vi "Filters.vi"() -> ()   [LabVIEW 2009]
uses:
  <vilib>/vision/NI_Vision_Development_Module.lvlib
panel:
  out "Filter Binary":T1(plugin-control)
  in  "file (use dialog)":path=path "C:/Documents and Settings/dgrieneisen/My Documents/Robotics/Athena/weights.fl"
  in  "Stop":bool
  in  "Filter Select":T2(radio)
  out "Filter Settings":T2(tab)
  in  "Red Range":cluster{"Lower value":i32, "Upper value":i32}={"Lower value"=120, "Upper value"=200}
  in  "Green Range":cluster{"Lower value":i32, "Upper value":i32}={"Lower value"=0, "Upper value"=255}
  in  "Blue Range":cluster{"Lower value":i32, "Upper value":i32}={"Lower value"=100, "Upper value"=255}
  in  "Color Mode":u16(ring) items=["RGB", "HSL", "HSV", "HSI"]
  in  "Hue Range":cluster{"Lower value":i32, "Upper value":i32}={"Lower value"=0, "Upper value"=255}
  in  "Saturation Range":cluster{"Lower value":i32, "Upper value":i32}={"Lower value"=0, "Upper value"=255}
  in  "Luma Range":cluster{"Lower value":i32, "Upper value":i32}={"Lower value"=0, "Upper value"=255}
  in  "Color Mode HSL":u16(ring)=1 items=["RGB", "HSL", "HSV", "HSI"]
  in  "Red Scalar":sgl=3.0
  in  "Green Scalar":sgl=3.0
  in  "Blue Scalar":sgl=3.3
  in  "Luma Scalar Low":sgl=4.0
  in  "Sat Scalar":sgl=2.5
  in  "Hue Scalar":sgl=5.0
  in  "Luma Scalar High":sgl=4.0
  in  "res/2":i32=3
  in  "Sample Rate":i32=3
  in  "ANN Level":dbl=0.5
  in  "ANN Out Switch":bool
  in  "Input Image Path":path=path "C:/Documents and Settings/dgrieneisen/My Documents/Robotics/Athena/image2004.jpg"
  out "'input Image":T1(plugin-control)
  out "Filtered Image":T1(plugin-control)
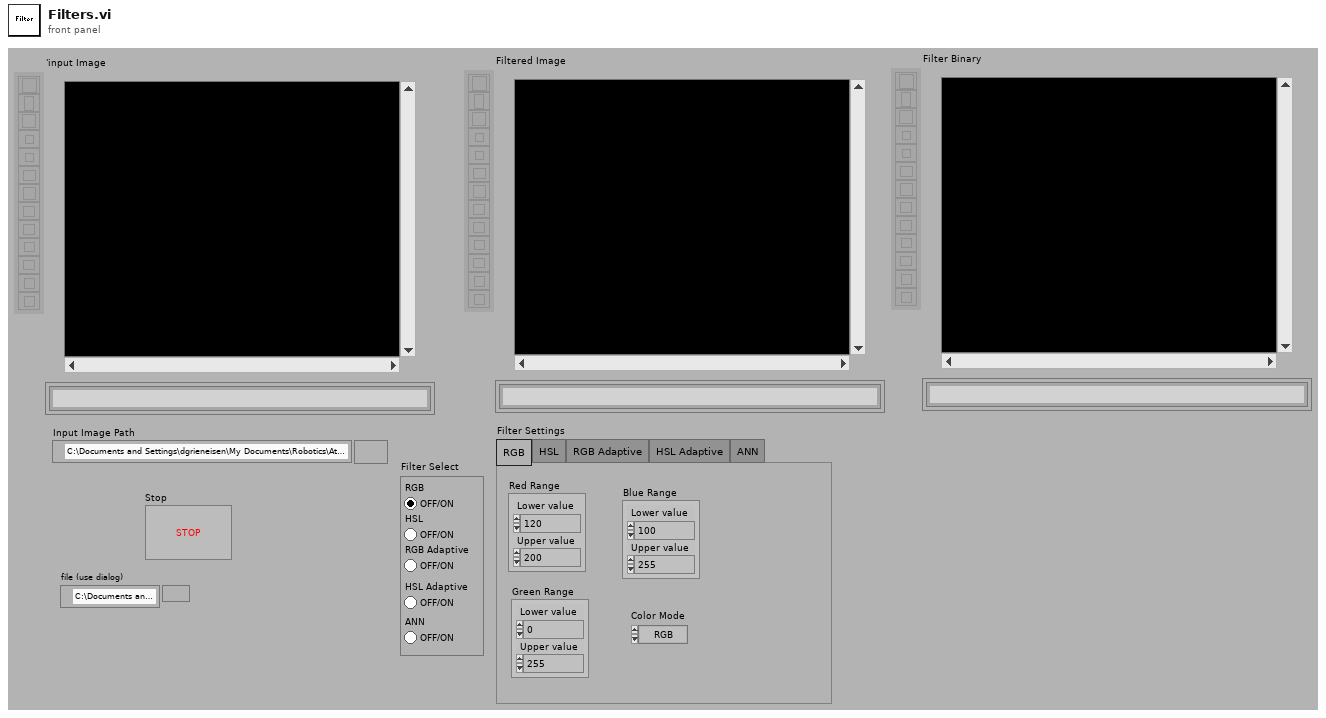
[diagram p1: front panel]
types:
  T1 = typedef "IMAQ Image.ctl" = refnum<image>
  T2 = enum32{"RGB", "HSL", "RGB Adaptive", "HSL Adaptive", "ANN"}
  T3 = typedef "Image Type" = u32
  T4 = cluster{"Num Hidden Layer":i32, "Function Final Layer":u16, "Function Hidden Layer":u16, dbl[], dbl[][]}
  T5 = cluster{"histogram":u32[], "Minimal Value":sgl, "Maximal Value":sgl, "Starting Value":sgl, "Interval Width":sgl, "Mean Value":sgl, "Standard  Variation":sgl, "Area (pixels)":i32}
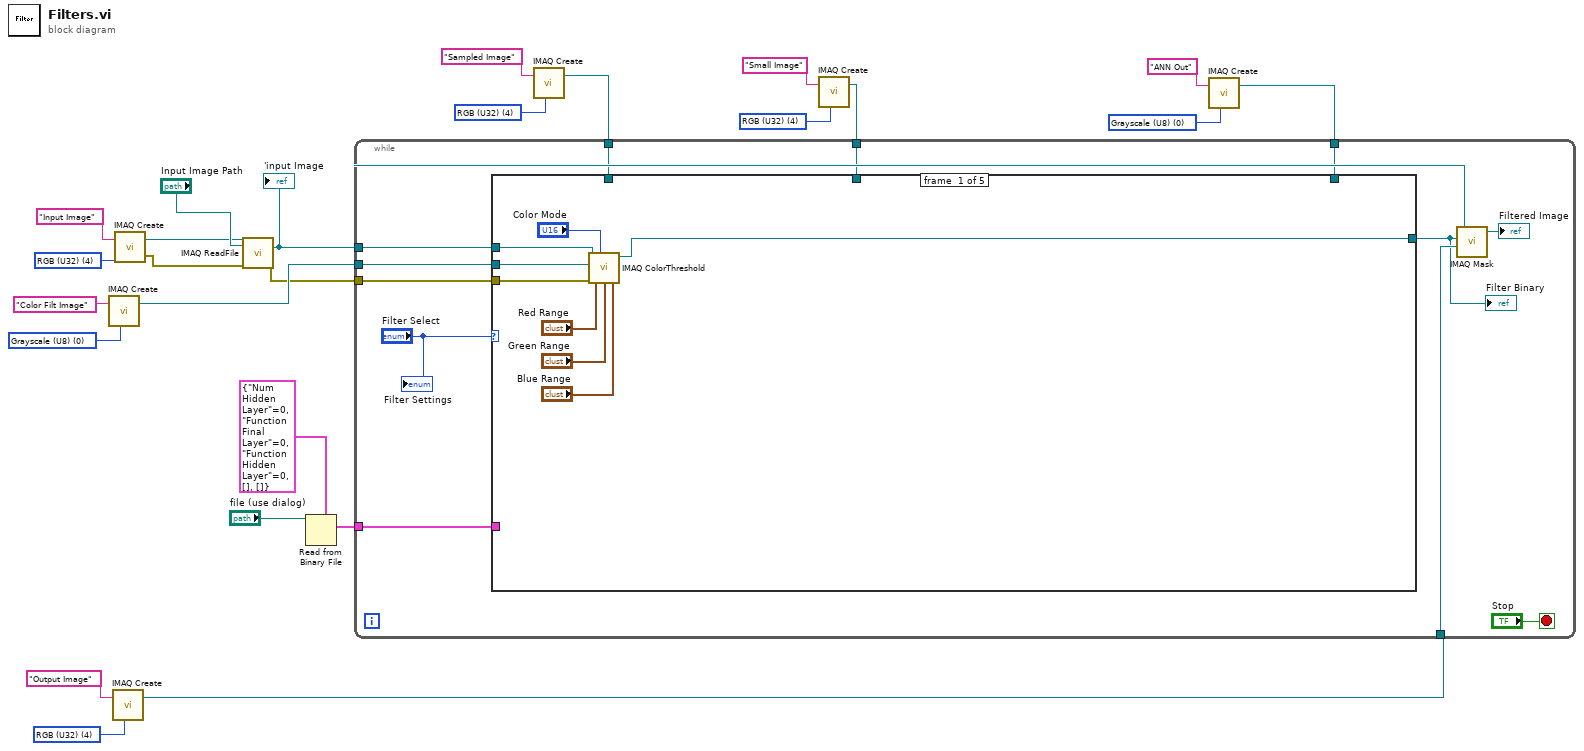
[diagram p0: block diagram]
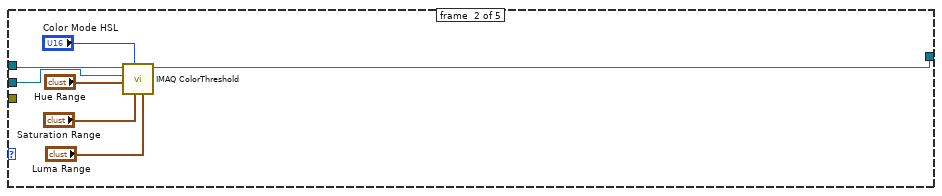
[diagram p2: hidden frame]
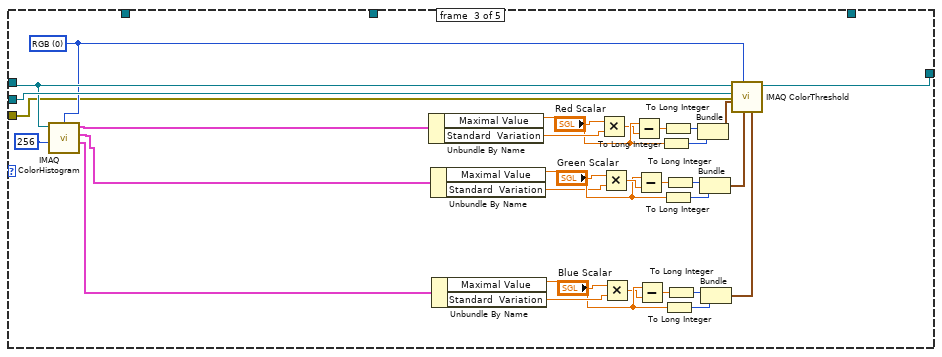
[diagram p3: hidden frame]
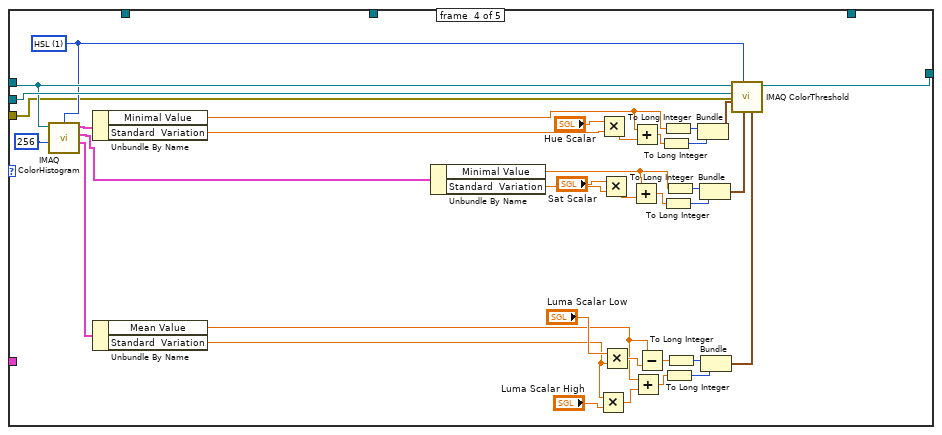
[diagram p4: hidden frame]
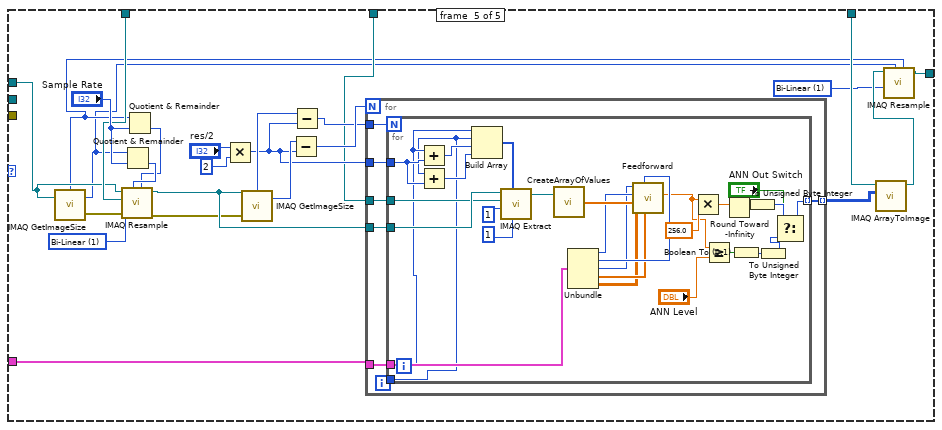
[diagram p5: hidden frame]
diagram:
  w4 = T3 0 items=["Grayscale (U8)", "Grayscale (I16)", "Grayscale (SGL)", "Complex (CSG)", "RGB (U32)", "HSL (U32)", "RGB (U64)", "Grayscale (U16)"] ("Image Type")
  w8 = T3 4 items=["Grayscale (U8)", "Grayscale (I16)", "Grayscale (SGL)", "Complex (CSG)", "RGB (U32)", "HSL (U32)", "RGB (U64)", "Grayscale (U16)"] ("Image Type")
  w12 = T3 4 items=["Grayscale (U8)", "Grayscale (I16)", "Grayscale (SGL)", "Complex (CSG)", "RGB (U32)", "HSL (U32)", "RGB (U64)", "Grayscale (U16)"] ("Image Type")
  w21 = T3 4 items=["Grayscale (U8)", "Grayscale (I16)", "Grayscale (SGL)", "Complex (CSG)", "RGB (U32)", "HSL (U32)", "RGB (U64)", "Grayscale (U16)"] ("Image Type")
  w23 = T3 0 items=["Grayscale (U8)", "Grayscale (I16)", "Grayscale (SGL)", "Complex (CSG)", "RGB (U32)", "HSL (U32)", "RGB (U64)", "Grayscale (U16)"] ("Image Type")
  w25 = T3 4 items=["Grayscale (U8)", "Grayscale (I16)", "Grayscale (SGL)", "Complex (CSG)", "RGB (U32)", "HSL (U32)", "RGB (U64)", "Grayscale (U16)"] ("Image Type")
  n1 = call "IMAQ Create"("Image Name"="Color Filt Image", "Image Type"=w23) -> ("New Image"=w17:T1)  [unwired: 2 in, 2 out]
  n2 = call "IMAQ Create"("Image Name"="Output Image", "Image Type"=w21) -> ("New Image"=w15:T1)  [unwired: 2 in, 2 out]
  n3 = call "IMAQ Create"("Image Name"="Input Image", "Image Type"=w25) -> ("New Image"=w14:T1, "error out"=w18:errorcluster)  [unwired: 2 in, 1 out]
  n4 = call "IMAQ ReadFile"("File Path"="Input Image Path", "error in (no error)"=w18, "Image"=w14) -> ("error out"=w16:errorcluster, "Image Out"=w13:T1)  [unwired: 4 in, 3 out]
  "'input Image" <- w13
  n5 = Read from Binary File(5:T4 {"Num Hidden Layer"=0, "Function Final Layer"=0, "Function Hidden Layer"=0, [], []} ("Cluster"), 11:"file (use dialog)") -> (2:w6:T4)  [unwired: 4 in, 3 out]
  n6 = call "IMAQ Create"("Image Name"="Sampled Image", "Image Type"=w12) -> ("New Image"=w10:T1)  [unwired: 2 in, 2 out]
  n7 = call "IMAQ Create"("Image Name"="Small Image", "Image Type"=w8) -> ("New Image"=w7:T1)  [unwired: 2 in, 2 out]
  n8 = call "IMAQ Create"("Image Name"="ANN Out", "Image Type"=w4) -> ("New Image"=w2:T1)  [unwired: 2 in, 2 out]
  n9 = while {
    tunnel: w17 -> [w37]
    tunnel: w16 -> [w36]
    tunnel: w15 -> [w35]
    tunnel: w13 -> [w33]
    tunnel: w10 -> [w30]
    tunnel: w7 -> [w29]
    tunnel: w6 -> [w28]
    tunnel: w2 -> [w27]
    stop <- "Stop" stop-if-true
    n10 = case shown="\"RGB\", Default" "Filter Select" {
      tunnel: w37 -> [w45 w50 w84 w120 _]
      tunnel: w36 -> [w44 _ w71 w110 _]
      tunnel: w33 -> [w40 w51 w83 w119 w130]
      tunnel: [w38 w46 w85 w121 w125] -> w26
      tunnel: w30 -> [_ _ _ _ w131]
      tunnel: w29 -> [_ _ _ _ w129]
      tunnel: w28 -> [_ _ _ _ w128]
      tunnel: w27 -> [_ _ _ _ w127]
      frame #0 {
        n11 = call "IMAQ ColorThreshold"("Blue or Luma or Val or Inten Range"="Blue Range", "Green or Sat Range"="Green Range", "Color Mode"="Color Mode", "error in (no error)"=w44, "Red or Hue Range"="Red Range", "Image Dst"=w45, "Image Src"=w40) -> ("Image Dst Out"=w38:T1)  [unwired: 3 in, 1 out]
      }
      frame #1 {
        n12 = call "IMAQ ColorThreshold"("Blue or Luma or Val or Inten Range"="Luma Range", "Green or Sat Range"="Saturation Range", "Color Mode"="Color Mode HSL", "Red or Hue Range"="Hue Range", "Image Dst"=w50, "Image Src"=w51) -> ("Image Dst Out"=w46:T1)  [unwired: 4 in, 1 out]
      }
      frame #2 {
        w81 = u16 0 items=["RGB", "HSL", "HSV", "HSI"] ("Color Mode")
        n13 = call "IMAQ ColorHistogram"("Color Mode"=w81, "Image Src"=w83, "Number of Classes"=256) -> ("Red or Hue or X or L* Histogram Report"=w80:T5, "Green or Sat or Y or a* Histogram Report"=w54:T5, "Blue or Luma or Val or Inten or Z or b* Histogram Report"=w53:T5)  [unwired: 3 in, 1 out]
        n14 = Unbundle By Name(w80) -> ("Maximal Value"=w74:sgl, "Standard  Variation"=w76:sgl)
        n15 = Unbundle By Name(w54) -> ("Maximal Value"=w68:sgl, "Standard  Variation"=w66:sgl)
        n16 = Unbundle By Name(w53) -> ("Maximal Value"=w59:sgl, "Standard  Variation"=w61:sgl)
        n17 = Multiply(x="Red Scalar", y=w76) -> (x*y=w73:sgl)
        n18 = Multiply(x="Green Scalar", y=w66) -> (x*y=w69:sgl)
        n19 = Multiply(x="Blue Scalar", y=w61) -> (x*y=w58:sgl)
        n20 = Subtract(x=w74, y=w73) -> (x-y=w75:sgl)
        n21 = Subtract(x=w68, y=w69) -> (x-y=w67:sgl)
        n22 = Subtract(x=w59, y=w58) -> (x-y=w60:sgl)
        n23 = To Long Integer(number=w74) -> (32bit integer=w77:i32)
        n24 = To Long Integer(number=w75) -> (32bit integer=w78:i32)
        n25 = To Long Integer(number=w68) -> (32bit integer=w65:i32)
        n26 = To Long Integer(number=w59) -> (32bit integer=w62:i32)
        n27 = To Long Integer(number=w67) -> (32bit integer=w64:i32)
        n28 = To Long Integer(number=w60) -> (32bit integer=w63:i32)
        n29 = Bundle(w78, w77) -> (w79:cluster{i32, i32})  [unwired: 1 in]
        n30 = Bundle(w64, w65) -> (w56:cluster{i32, i32})  [unwired: 1 in]
        n31 = Bundle(w63, w62) -> (w55:cluster{i32, i32})  [unwired: 1 in]
        n32 = call "IMAQ ColorThreshold"("Blue or Luma or Val or Inten Range"=w55, "Green or Sat Range"=w56, "Color Mode"=w81, "error in (no error)"=w71, "Red or Hue Range"=w79, "Image Dst"=w84, "Image Src"=w83) -> ("Image Dst Out"=w85:T1)  [unwired: 3 in, 1 out]
      }
      frame #3 {
        w117 = u16 1 items=["RGB", "HSL", "HSV", "HSI"] ("Color Mode")
        n33 = call "IMAQ ColorHistogram"("Color Mode"=w117, "Image Src"=w119, "Number of Classes"=256) -> ("Red or Hue or X or L* Histogram Report"=w116:T5, "Green or Sat or Y or a* Histogram Report"=w100:T5, "Blue or Luma or Val or Inten or Z or b* Histogram Report"=w99:T5)  [unwired: 3 in, 1 out]
        n34 = Unbundle By Name(w116) -> ("Minimal Value"=w97:sgl, "Standard  Variation"=w112:sgl)
        n35 = Unbundle By Name(w99) -> ("Mean Value"=w87:sgl, "Standard  Variation"=w90:sgl)
        n36 = Unbundle By Name(w100) -> ("Minimal Value"=w95:sgl, "Standard  Variation"=w108:sgl)
        n37 = Multiply(x=w90, y="Luma Scalar High") -> (x*y=w88:sgl)
        n38 = Multiply(x="Hue Scalar", y=w112) -> (x*y=w98:sgl)
        n39 = Multiply(x="Sat Scalar", y=w108) -> (x*y=w94:sgl)
        n40 = Multiply(x="Luma Scalar Low", y=w90) -> (x*y=w103:sgl)
        n41 = Add(x=w95, y=w94) -> (x+y=w93:sgl)
        n42 = Add(x=w97, y=w98) -> (x+y=w96:sgl)
        n43 = Add(x=w87, y=w88) -> (x+y=w89:sgl)
        n44 = Subtract(x=w87, y=w103) -> (x-y=w104:sgl)
        n45 = To Long Integer(number=w96) -> (32bit integer=w113:i32)
        n46 = To Long Integer(number=w97) -> (32bit integer=w114:i32)
        n47 = To Long Integer(number=w93) -> (32bit integer=w107:i32)
        n48 = To Long Integer(number=w89) -> (32bit integer=w86:i32)
        n49 = To Long Integer(number=w95) -> (32bit integer=w106:i32)
        n50 = To Long Integer(number=w104) -> (32bit integer=w105:i32)
        n51 = Bundle(w114, w113) -> (w115:cluster{i32, i32})  [unwired: 1 in]
        n52 = Bundle(w106, w107) -> (w102:cluster{i32, i32})  [unwired: 1 in]
        n53 = Bundle(w105, w86) -> (w101:cluster{i32, i32})  [unwired: 1 in]
        n54 = call "IMAQ ColorThreshold"("Blue or Luma or Val or Inten Range"=w101, "Green or Sat Range"=w102, "Color Mode"=w117, "error in (no error)"=w110, "Red or Hue Range"=w115, "Image Dst"=w120, "Image Src"=w119) -> ("Image Dst Out"=w121:T1)  [unwired: 3 in, 1 out]
      }
      frame #4 {
        w124 = u32 1 items=["Zero Order", "Bi-Linear", "Quadratic", "Cubic Spline"] ("Interpolation Type")
        w142 = u32 1 items=["Zero Order", "Bi-Linear", "Quadratic", "Cubic Spline"] ("Interpolation Type")
        n55 = call "IMAQ GetImageSize"("Image"=w130) -> ("Y Resolution"=w122:i32, "X Resolution"=w123:i32, "error out"=w146:errorcluster)  [unwired: 3 in]
        n56 = Quotient & Remainder(x=w122, y="Sample Rate") -> (floor(x/y)=w145:i32)  [unwired: 1 out]
        n57 = Quotient & Remainder(x=w123, y="Sample Rate") -> (floor(x/y)=w144:i32)  [unwired: 1 out]
        n58 = call "IMAQ Resample"("X Resolution"=w144, "Y Resolution"=w145, "error in (no error)"=w146, "Interpolation Type"=w142, "Image Dst"=w131, "Image Src"=w130) -> ("error out"=w132:errorcluster, "Image Dst Out"=w136:T1)  [unwired: 4 in]
        n59 = Multiply(x="res/2", y=2) -> (x*y=w137:i32)
        n60 = call "IMAQ GetImageSize"("Image"=w136, "error in (no error)"=w132) -> ("Y Resolution"=w141:i32, "X Resolution"=w138:i32)  [unwired: 2 in, 1 out]
        n61 = Subtract(x=w141, y=w137) -> (x-y=w134:i32)
        n62 = Subtract(x=w138, y=w137) -> (x-y=w133:i32)
        n63 = for {
          N: w134 -> [_]
          tunnel: w137 -> [w153]
          tunnel: w136 -> [w152]
          tunnel: w128 -> [w151]
          tunnel: [w150] -> w135 mode=indexing
          tunnel: w129 -> [w149]
          tunnel: w133 -> [w148]
          i -> [w147]
          n64 = for {
            N: w148 -> [_]
            tunnel: w153 -> [w179]
            tunnel: w152 -> [w177]
            tunnel: w151 -> [w174]
            tunnel: [w155] -> w150 mode=indexing
            tunnel: w149 -> [w168]
            tunnel: w147 -> [w164]
            i -> [w165]
            n65 = Add(x=w165, y=w179) -> (x+y=w181:i32)
            n66 = Add(x=w164, y=w179) -> (x+y=w180:i32)
            n67 = Build Array(w165, w164, w181, w180) -> (w178:i32[])
            n68 = call "IMAQ Extract"("Y Step Size"=1, "Optional Rectangle"=w178, "X Step Size"=1, "Image Dst"=w168, "Image Src"=w177) -> ("Image Dst Out"=w176:T1)  [unwired: 1 in, 5 out]
            n69 = call "CreateArrayOfValues.vi"("Image Out"=w176) -> ("Array"=w175:dbl[])  [unwired: 1 in]
            n70 = Unbundle(w174) -> ("Num Hidden Layer"=w173:i32, "Function Final Layer"=w172:u16, "Function Hidden Layer"=w171:u16, w170:dbl[], w169:dbl[][])
            n71 = call "Feedforward.vi"("Final Weights"=w170, "Function Final Layer"=w172, "Hidden Weights"=w169, "Inputs"=w175, "Num Hidden Layer"=w173, "Function Hidden Layer"=w171) -> ("Output"=w160:dbl)  [unwired: 3 out]
            n72 = Multiply(x=w160, y=256.0) -> (x*y=w166:dbl)
            n73 = Greater Or Equal?(x=w160, y="ANN Level") -> (x >= y?=w162:bool)
            n74 = Round Toward -Infinity(1:w166) -> (0:w159:dbl)
            n75 = Boolean To (0,1)(Boolean=w162) -> (0, 1=w158:i16)
            n76 = To Unsigned Byte Integer(number=w159) -> (unsigned 8bit integer=w156:u8)
            n77 = To Unsigned Byte Integer(number=w158) -> (unsigned 8bit integer=w157:u8)
            n78 = Select(t=w156, s="ANN Out Switch", f=w157) -> (s? t:f=w155:u8)
          }
        }
        n79 = call "IMAQ ArrayToImage"("Image Pixels (U8)"=w135, "Image"=w127) -> ("Image Out"=w126:T1)  [unwired: 8 in, 1 out]
        n80 = call "IMAQ Resample"("X Resolution"=w123, "Y Resolution"=w122, "Interpolation Type"=w124, "Image Src"=w126) -> ("Image Dst Out"=w125:T1)  [unwired: 6 in, 1 out]
      }
    }
    "Filter Binary" <- w26
    n81 = call "IMAQ Mask"("Image Dst"=w35, "Image Mask"=w26, "Image Src"=w33) -> ("Image Dst Out"=→"Filtered Image":T1)  [unwired: 2 in, 1 out]
    "Filter Settings" <- "Filter Select"
  }
